vi "OPO_Send_Value.vi"(8 "error in (no error)":errorcluster, 10 "Loop":i16=1 min=1, 11 "OPO Inputs":T1={"OPO AutoAlignment ON"=FALSE, "OPO Start Value"=210.0, "OPO Stop Value"=270.0, "OPO Step"=30.0} {"OPO Step" min=1.0 max=60.0; "OPO Stop Value" min=210.0 max=270.0; "OPO Start Value" min=210.0 max=270.0}) -> (0 "error out":errorcluster, 3 "OPO Value":i16)   [LabVIEW 2024]
doc: "This VI calculates the next value of the OPO and send it to the PC-OPO via the network with TCP/IP protocol.\nThe IP address of the TCP/IP client is read from the PIL.ini file.\nThe TCP/IP client should have been already started on PC-OPO."
uses:
  controls/OPO_Inputs.ctl
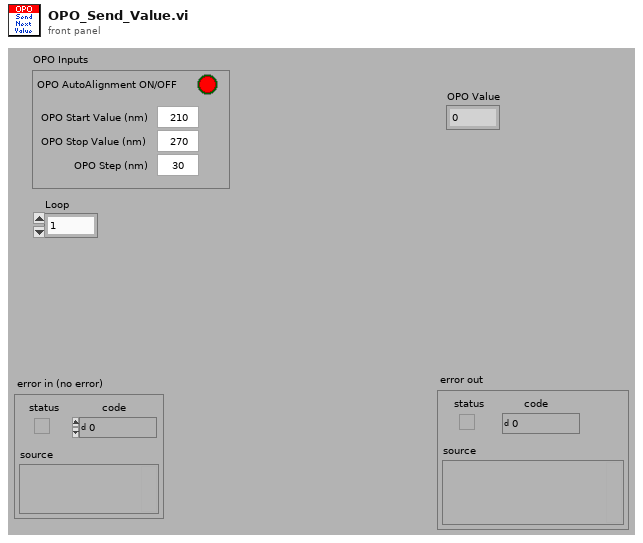
[diagram p1: front panel]
types:
  T1 = typedef "OPO_Inputs.ctl" = cluster{"OPO AutoAlignment ON":bool, "OPO Start Value":dbl, "OPO Stop Value":dbl, "OPO Step":dbl}
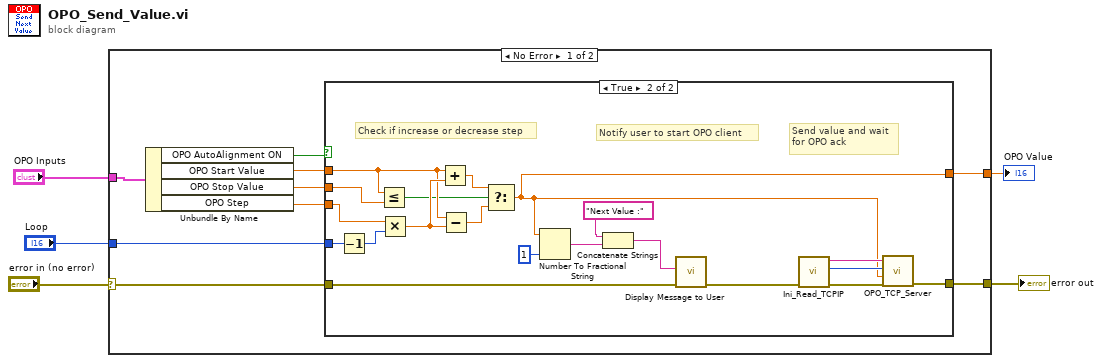
[diagram p0: block diagram]
diagram:
  n1 = case shown="No Error" "error in (no error)" {
    selector: "error in (no error)" -> [w14 w36]
    tunnel: [w9 w36] -> w5
    tunnel: "OPO Inputs" -> [w13 _]
    tunnel: "Loop" -> [w10 _]
    tunnel: [w8 _] -> w1
    frame No Error {
      n2 = Unbundle By Name(w13) -> ("OPO AutoAlignment ON"=w7:bool, "OPO Start Value"=w11:dbl, "OPO Stop Value"=w6:dbl, "OPO Step"=w12:dbl)
      n3 = case shown="True" w7 {
        tunnel: w14 -> [w15 w32]
        tunnel: w12 -> [_ w31]
        tunnel: w11 -> [_ w21]
        tunnel: w10 -> [_ w30]
        tunnel: [w15 w27] -> w9
        tunnel: [_ w17] -> w8
        tunnel: w6 -> [_ w23]
        frame False {
        }
        frame True {
          # "Notify user to start OPO client"
          # "Check if increase or decrease step"
          # "Send value and wait\nfor OPO ack"
          n4 = Decrement(x=w30) -> (x-1=w24:i16)
          n5 = Less Or Equal?(x=w21, y=w23) -> (x <= y?=w20:bool)
          n6 = Multiply(x=w31, y=w24) -> (x*y=w22:dbl)
          n7 = Add(x=w21, y=w22) -> (x+y=w19:dbl)
          n8 = Subtract(x=w21, y=w22) -> (x-y=w18:dbl)
          n9 = Select(t=w19, s=w20, f=w18) -> (s? t:f=w17:dbl)
          n10 = Number To Fractional String(number=w17, precision (6)=i16 1) -> (F-format string=w35:string)  [unwired: 2 in]
          n11 = Concatenate Strings("Next Value :" ("string"), w35) -> (w33:string)
          n12 = call "Display Message to User"("error in (no error)"=w32, "Message"=w33) -> ("error out"=w29:errorcluster)  [unwired: 8 in, 1 out]
          n13 = call "Ini_Read_TCPIP.vi"("error in (no error)"=w29) -> ("error out"=w28:errorcluster, "port"=w25:u16, "address"=w26:string)  [unwired: 7 in]
          n14 = call "OPO_TCP_Server.vi"("address"=w26, "port"=w25, "OPO Value"=w17, "error in (no error)"=w28) -> ("error out"=w27:errorcluster)  [unwired: 6 in]
        }
      }
    }
    frame Error {
    }
  }
  "error out" <- w5
  "OPO Value" <- w1
